vi "Example Main Program.vi"() -> ()   [LabVIEW 2018]
uses:
  <vilib>/Platform/TimedLoop/XDataNode/timing_clust.ctl
  <vilib>/Platform/TimedLoop/XDataNode/nitl_modes.ctl
  <vilib>/Platform/TimedLoop/XDataNode/wakeup.ctl
  <vilib>/Utility/file.llb/Read Delimited Spreadsheet (DBL).vi
  <vilib>/platform/TimedLoop/XDataNode/XDataNode.xnode
  COBRA Gait Phase Estimation Library.lvlib
  <vilib>/Platform/TimedLoop/XDataNode/XDNodeRunTimeDep.lvlib
panel:
  out "Waveform Chart 3":dbl(graph)
  out "Waveform Chart 2":dbl(graph)
  in  "Stop":bool
  out "Waveform Chart":dbl(graph)
  in  "file path (dialog if empty)":path
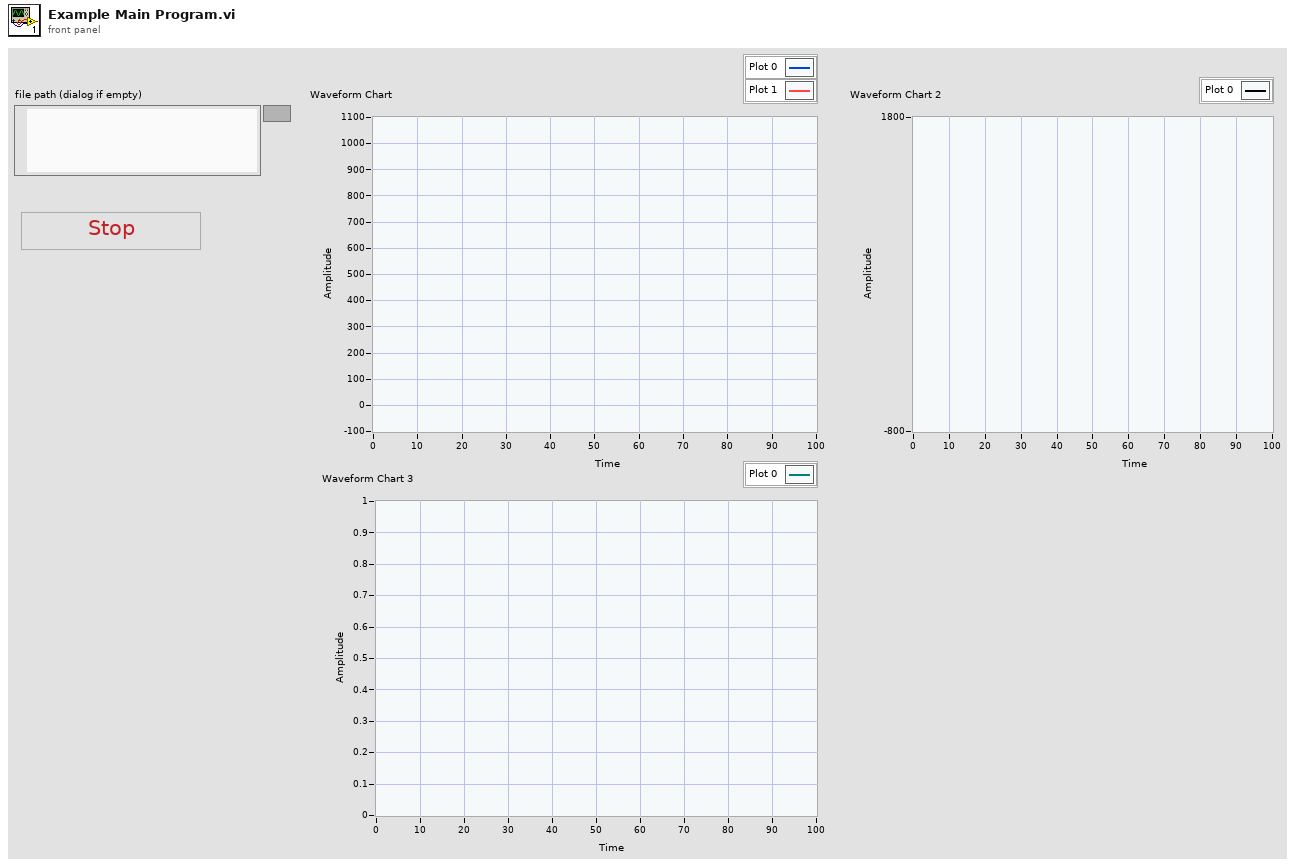
[diagram p1: front panel]
types:
  T1 = typedef "XDNodeRunTimeDep.lvlib/timing_clust.ctl" = cluster{"Expected End [f-1]":u64, "Actual End [f-1]":u64, "Finished Late? [f-1]":bool, "Expected End [i-1]":u64, "Actual End [i-1]":u64, "Finished Late? [i-1]":bool, "Expected Start [i]":u64, "Actual Start [i]":u64, "Expected Start [f]":u64, "Actual Start [f]":u64, "Source Name":string, "Structure Name":string, "Period":i64, "Deadline":i64, "Offset":i64, "Start":i64, "Priority":i32, "Timeout":i32, "Mode":T2, "Wakeup Reason":T3, "Error":errorcluster, "Source Type":string, "Secondary Source Type":string, "Global End Time":u64, "Global Start Time":u64, "Frame Duration":u64, "Iteration Duration":u64, "Assigned CPU":i32, "I/O Scan Engine Mode":u32}
  T2 = typedef "XDNodeRunTimeDep.lvlib/nitl_modes.ctl" = enum32{"No Change", "Process missed periods, maintain original phase", "Discard missed periods, maintain original phase", "Process missed periods, ignore original phase", "Discard missed periods, ignore original phase"}
  T3 = typedef "XDNodeRunTimeDep.lvlib/wakeup.ctl" = enum32{"Normal", "Aborted", "Asynchronous wakeup", "Timing source error", "Timed loop error", "Timeout"}
  T4 = cluster{"Saturation Threshold":dbl, "LP Filter Cutoff\nFrequency":dbl, "HS Force Rate Threshold":dbl, "Sampling Frequency (Hz)":dbl, "Wait Window (s)":dbl}
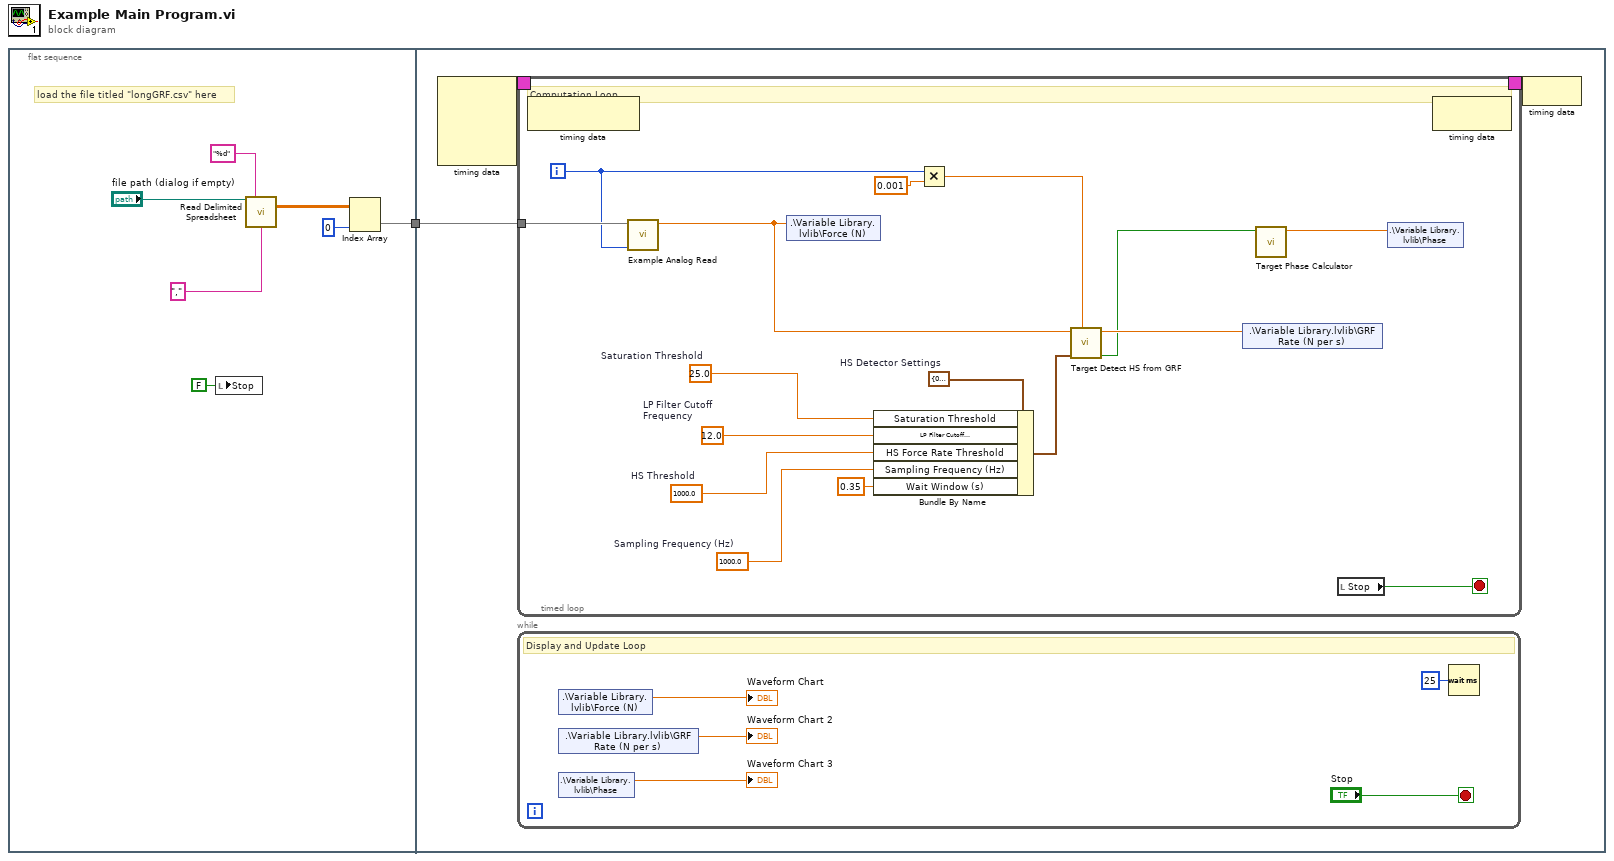
[diagram p0: block diagram]
diagram:
  n1 = flat-sequence {
    tunnel: [w3] -> w1
    tunnel: w1 -> [w11]
    frame #0 {
      # "load the file titled \"longGRF.csv\" here"
      n2 = local write "Stop"(FALSE ("Stop")) -> ()
      n3 = call-poly <vilib>:"Read Delimited Spreadsheet.vi"("file path (dialog if empty)"="file path (dialog if empty)", "format (%.3f)"="%d", "delimiter (\\t)"="," ("delimiter (\\t)")) -> ("all rows"=w5:dbl[][])  [unwired: 7 in, 5 out]
      n4 = Index Array "Index Array"(array=w5, index (col)=0 ("disabled index (col)")) -> (element=w3:dbl[])  [unwired: 1 in]
    }
    frame #1 {
      n5 = node-c288() -> (w10:T1)  [unwired: 4 in]
      n6 = timed-loop {
        tunnel: w11 -> [w26]
        timing: w10 -> [_]
        timing-out: [_] -> w9
        i -> [w21]
        stop <- w27 stop-if-true
        w14 = 1000.0  # Sampling Frequency (Hz)
        w15 = 1000.0  # HS Threshold
        w16 = 12.0  # LP Filter Cutoff Frequency
        w17 = 25.0  # Saturation Threshold
        w19 = T4 {"Saturation Threshold"=0.0, "LP Filter Cutoff\nFrequency"=12.0, "HS Force Rate Threshold"=0.0, "Sampling Frequency (Hz)"=0.0, "Wait Window (s)"=0.0}  # HS Detector Settings
        # "Computation Loop"
        n7 = node-c288() -> ()  [unwired: 1 in, 1 out]
        n8 = call "Example Analog Read.vi"("Index"=w21, "Array"=w26) -> ("Force (N)"=w23:dbl)  [unwired: 9 in]
        n9 = shared-variable ".\\Variable Library.lvlib\\Force (N)"(w23) -> ()  [unwired: 1 in, 1 out]
        n10 = Bundle By Name(cluster=w19, "Saturation Threshold"=w17, "LP Filter Cutoff\nFrequency"=w16, "HS Force Rate Threshold"=w15, "Sampling Frequency (Hz)"=w14, "Wait Window (s)"=0.35) -> (w18:T4)
        n11 = Multiply(x=w21, y=0.001) -> (x*y=w20:dbl)
        n12 = call "Target Detect HS from GRF.vi"("Main Clock Line (s)"=w20, "HS Detector Settings"=w18, "Fz"=w23) -> ("HS"=w12:bool, "GRF Rate (N/s)"=w25:dbl)  [unwired: 6 in, 1 out]
        n13 = shared-variable ".\\Variable Library.lvlib\\GRF Rate (N per s)"(w25) -> ()  [unwired: 1 in, 1 out]
        n14 = call "Target Phase Calculator.vi"("HS Detected"=w12) -> ("Phase"=w24:dbl)  [unwired: 10 in]
        n15 = local read "Stop"() -> (w27:bool)
        n16 = shared-variable ".\\Variable Library.lvlib\\Phase"(w24) -> ()  [unwired: 1 in, 1 out]
        n17 = node-c288() -> ()  [unwired: 1 in, 1 out]
      }
      n18 = while {
        stop <- "Stop" stop-if-true
        # "Display and Update Loop"
        n19 = shared-variable ".\\Variable Library.lvlib\\Force (N)"() -> (→"Waveform Chart":dbl)  [unwired: 1 in, 1 out]
        n20 = shared-variable ".\\Variable Library.lvlib\\GRF Rate (N per s)"() -> (→"Waveform Chart 2":dbl)  [unwired: 1 in, 1 out]
        n21 = shared-variable ".\\Variable Library.lvlib\\Phase"() -> (→"Waveform Chart 3":dbl)  [unwired: 1 in, 1 out]
        n22 = Wait (ms)(milliseconds to wait=u32 25) -> ()  [unwired: 1 out]
      }
      n23 = node-c288(w9) -> ()
    }
  }
